vi "Flush Serial - host.vi"(9 "Timeout (ms)":i32=100, 11 "Refnum in":refnum<k20>) -> (3 "Reference Out":refnum<k20>)   [LabVIEW 2012]
uses:
  <vilib>/Utility/error.llb/Error Cluster From Error Code.vi
  <vilib>/rvi/errors/niLvFpgaAdjustHostInterfaceError.vi
  <vilib>/rvi/interface/nirviMethod/nirviMethod.xnode
  <vilib>/FPGAPlugInAG/Dynamic/niLvFpga_ReadFifo_Dynamic.vi
  <vilib>/rvi/errors/niLvFpgaMergeErrorWithErrorCode.vi
panel:
  out "Data":u8[](array[numeric])
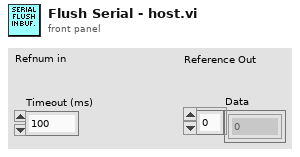
[diagram p1: front panel]
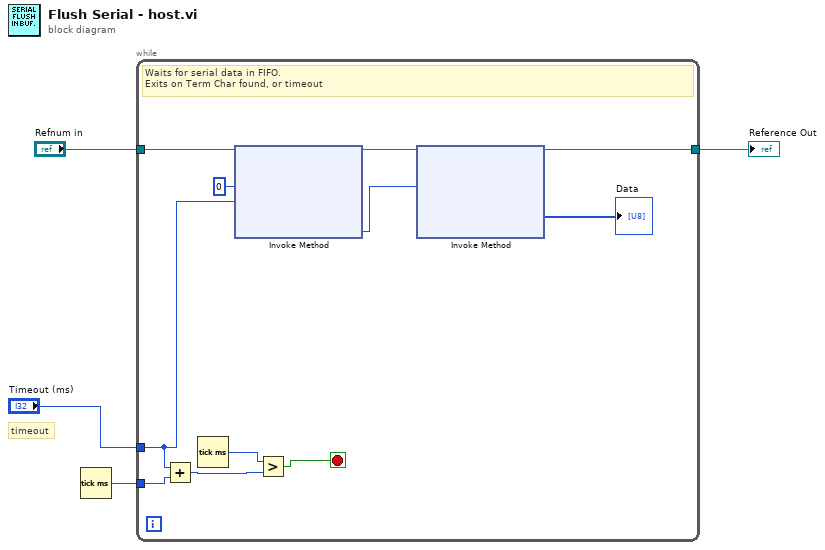
[diagram p0: block diagram]
diagram:
  # "timeout"
  n1 = Tick Count (ms)() -> (millisecond timer value=w2:u32)
  n2 = while {
    tunnel: "Refnum in" -> [w12]
    tunnel: "Timeout (ms)" -> [w11]
    tunnel: w2 -> [w14]
    tunnel: [w9] -> w1
    stop <- w6 stop-if-true
    # "Waits for serial data in FIFO.\nExits on Term Char found, or timeout"
    n3 = Add(x=w11, y=w14) -> (x+y=w13:u32)
    n4 = Tick Count (ms)() -> (millisecond timer value=w15:u32)
    n5 = xnode "Invoke Method"("FPGA VI Reference In"=w12, "Number of Elements"=u32 0, "Timeout (ms)"=w11) -> ("FPGA VI Reference Out"=w10:refnum<k20>, "Elements Remaining"=w8:u32)  [unwired: 1 in, 2 out]
    n6 = Greater?(x=w15, y=w13) -> (0:w6:bool)
    n7 = xnode "Invoke Method"("FPGA VI Reference In"=w10, "Number of Elements"=w8) -> ("FPGA VI Reference Out"=w9:refnum<k20>, "Data"=→"Data":u8[])  [unwired: 2 in, 2 out]
  }
  "Reference Out" <- w1
